vi "Add Section to CFG File.vi"(8 "error in":errorcluster, 11 "Config in":refnum<class "Config.lvclass">) -> (0 "error out":errorcluster, 3 "Config out":refnum<class "Config.lvclass">)   [LabVIEW 2023, in "Config.lvlib" / "Config.lvclass"]
uses:
  Config.lvclass
  Config.lvclass/Config.ctl
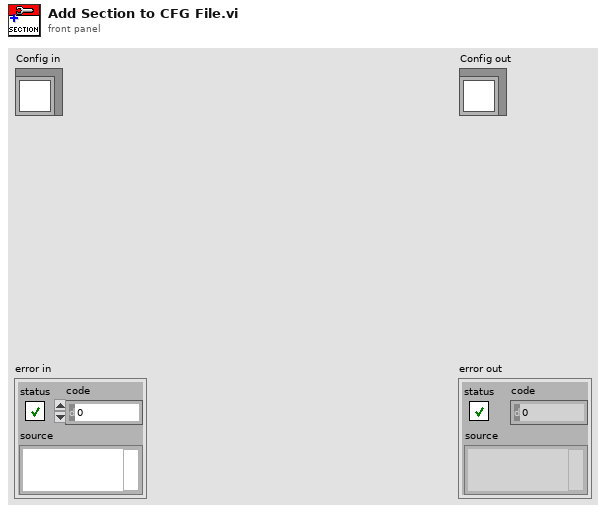
[diagram p1: front panel]
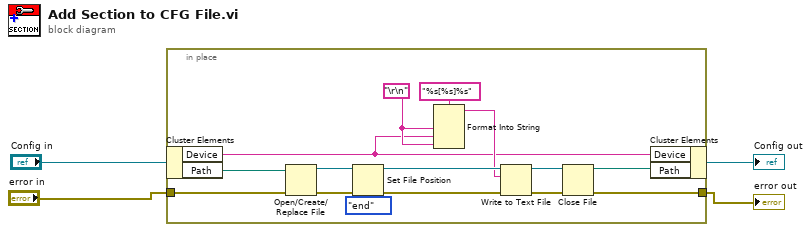
[diagram p0: block diagram]
diagram:
  n1 = in-place {
    in-place-border: [w11] -> w3
    in-place-border: "error in" -> [w10]
    w8 = "\r\n"
    n2 = in-place-cluster #1("Config in") -> ("Device"=w5:string, "Path"=w19:path)
    n3 = Open/Create/Replace File(file path (use dialog)=w19, error in=w10) -> (refnum out=w18:refnum<file>, error out=w14:errorcluster)  [unwired: 4 in, 1 out]
    n4 = Set File Position(refnum=w18, from (0:start)=enum16{"start", "end", "current"}."end", error in=w14) -> (refnum out=w17:refnum<file>, error out=w13:errorcluster)  [unwired: 1 in]
    n5 = Format Into String(format string="%s[%s]%s", w8, w5, w8) -> (resulting string=w7:string)  [unwired: 2 in, 1 out]
    n6 = Write to Text File(file (use dialog)=w17, text=w7, error in=w13) -> (refnum out=w16:refnum<file>, error out=w12:errorcluster)  [unwired: 1 in, 1 out]
    n7 = Close File(refnum=w16, error in=w12) -> (path=w15:path, error out=w11:errorcluster)
    n8 = in-place-cluster #1("Device"=w5, "Path"=w15) -> (→"Config out":refnum<class "Config.lvclass">)
  }
  "error out" <- w3
